vi "Convert_allChannelProperties_to_JSON.vi"(8 "error in (no error)":errorcluster, 11 "allChannelProperties":T1 {"channel" min=1 max=8 step=1}) -> (0 "error out":errorcluster, 3 "<JSON>":string)   [LabVIEW 2019, in "Inst.KH7008.lvlib" / "Inst.Krohn-Hite-7008.lvclass"]
uses:
  Inst.Krohn-Hite-7008.lvclass
  KH7008/typedefs/allChannelProperties--Array.ctl
  KH7008/typedefs/channelProperties--Cluster.ctl
  KH7008/typedefs/channel--numeric.ctl
  KH7008/typedefs/gain--enum.ctl
  KH7008/typedefs/Input--Enum.ctl
  KH7008/typedefs/shunt--enum.ctl
  KH7008/typedefs/couple--Enum.ctl
  KH7008/typedefs/Filter--Enum.ctl
  3cd287df-e11a-49e5-8b51-e9e2427607d6.vi
  <vilib>/JDP Science/JSONtext/Variant to JSON Text.vi
  <vilib>/JDP Science/JSONtext/LVClass Serializer/JSONtext LVClass Serializer.lvclass
  <vilib>/JDP Science/JSONtext/JSONtext.lvlib
  KH7008/KH7008.lvlib
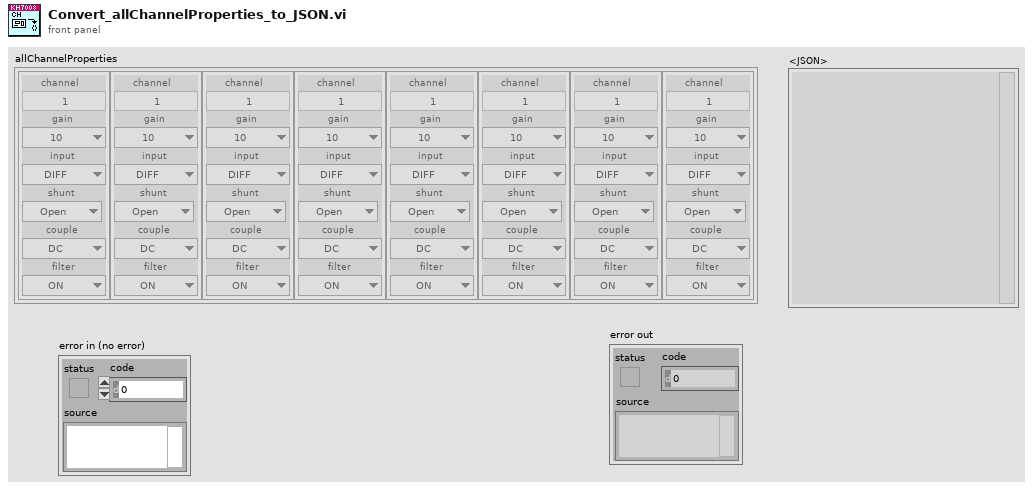
[diagram p1: front panel]
types:
  T1 = typedef "KH7008.lvlib/allChannelProperties--Array.ctl" = T2[]
  T2 = typedef "KH7008.lvlib/channelProperties--Cluster.ctl" = cluster{"channel":T3, "gain":T4, "input":T5, "shunt":T6, "couple":T7, "filter":T8}
  T3 = typedef "KH7008.lvlib/channel--numeric.ctl" = u16
  T4 = typedef "KH7008.lvlib/gain--enum.ctl" = enum16{"1", "10", "100", "1000"}
  T5 = typedef "KH7008.lvlib/input--enum.ctl" = enum16{"OFF", "SE+", "SE-", "DIFF"}
  T6 = typedef "KH7008.lvlib/shunt--enum.ctl" = enum16{"Open", "50", "500", "5k", "50k", "10M"}
  T7 = typedef "KH7008.lvlib/couple--enum.ctl" = enum16{"AC", "DC"}
  T8 = typedef "KH7008.lvlib/filter--enum.ctl" = enum16{"OFF", "ON"}
  T9 = typedef "Inst.KH7008.lvlib/Inst.Krohn-Hite-7008.lvclass/getAllChannelsDatabase--Cluster.ctl" = cluster{"device_id":string, "channel":u32, "gain":string, "input":string, "shunt":string, "couple":string, "filter":string}
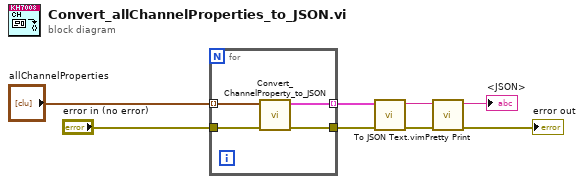
[diagram p0: block diagram]
diagram:
  n1 = for {
    tunnel: "allChannelProperties" -> [w12] mode=indexing
    tunnel: [w11] -> w8 mode=indexing
    tunnel: "error in (no error)" -> [w10]
    tunnel: [w9] -> w3
    n2 = call "Convert_ChannelProperty_to_JSON.vi"("error in (no error)"=w10, "channelProperties"=w12) -> ("error out"=w9:errorcluster, "getChannelResponse"=w11:T9)  [unwired: 8 in]
  }
  n3 = call "To JSON Text.vim"("error in (no error)"=w3, "Anything"=w8) -> ("error out"=w2:errorcluster, "<JSON>"=w6:string)  [unwired: 8 in]
  n4 = call <vilib>:"Pretty Print.vi"("error in (no error)"=w2, "JSON"=w6) -> ("error out"=→"error out":errorcluster, "<JSON>"=→"<JSON>":string)  [unwired: 7 in, 1 out]
